vi "P6 main start.vi"() -> ()   [LabVIEW 2016]
doc: "This is the main vi for the C(T) experiment, which measures the capacitance of a ferroelectric capacitor for a defined set of temperatures.\n\nPaul K Dixon\nPhysics 350\nCSUSB Physics"
uses:
  globals/C(T) global variables.vi
  C(T) subvis/temp control/globals/temp control global variables.vi
panel:
  in  "Def Set":dbl=30.0 caption="Default Setpoint (C)" format="%.2f"
  in  "Forced Stop":bool
  # "C(T) Experiment Main"
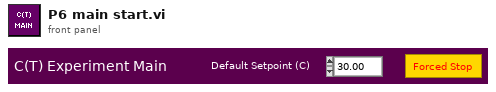
[diagram p1: front panel]
types:
  T1 = typedef "control parameters.ctl" = cluster{"Setpoint":dbl, "Control bandwidth":dbl, "Settle bandwidth":dbl, "Integral time":dbl, "Int\non":bool, "Derivative time":dbl, "Der\non":bool, "Settle time":dbl}
  T2 = cluster{"N cycles for averaging":i32, "N points per measurment":i32, "Measurment time interval":dbl}
  T3 = cluster{"N cycles for averaging":i32, "N points per measurement":i32, "Measurment time interval":dbl}
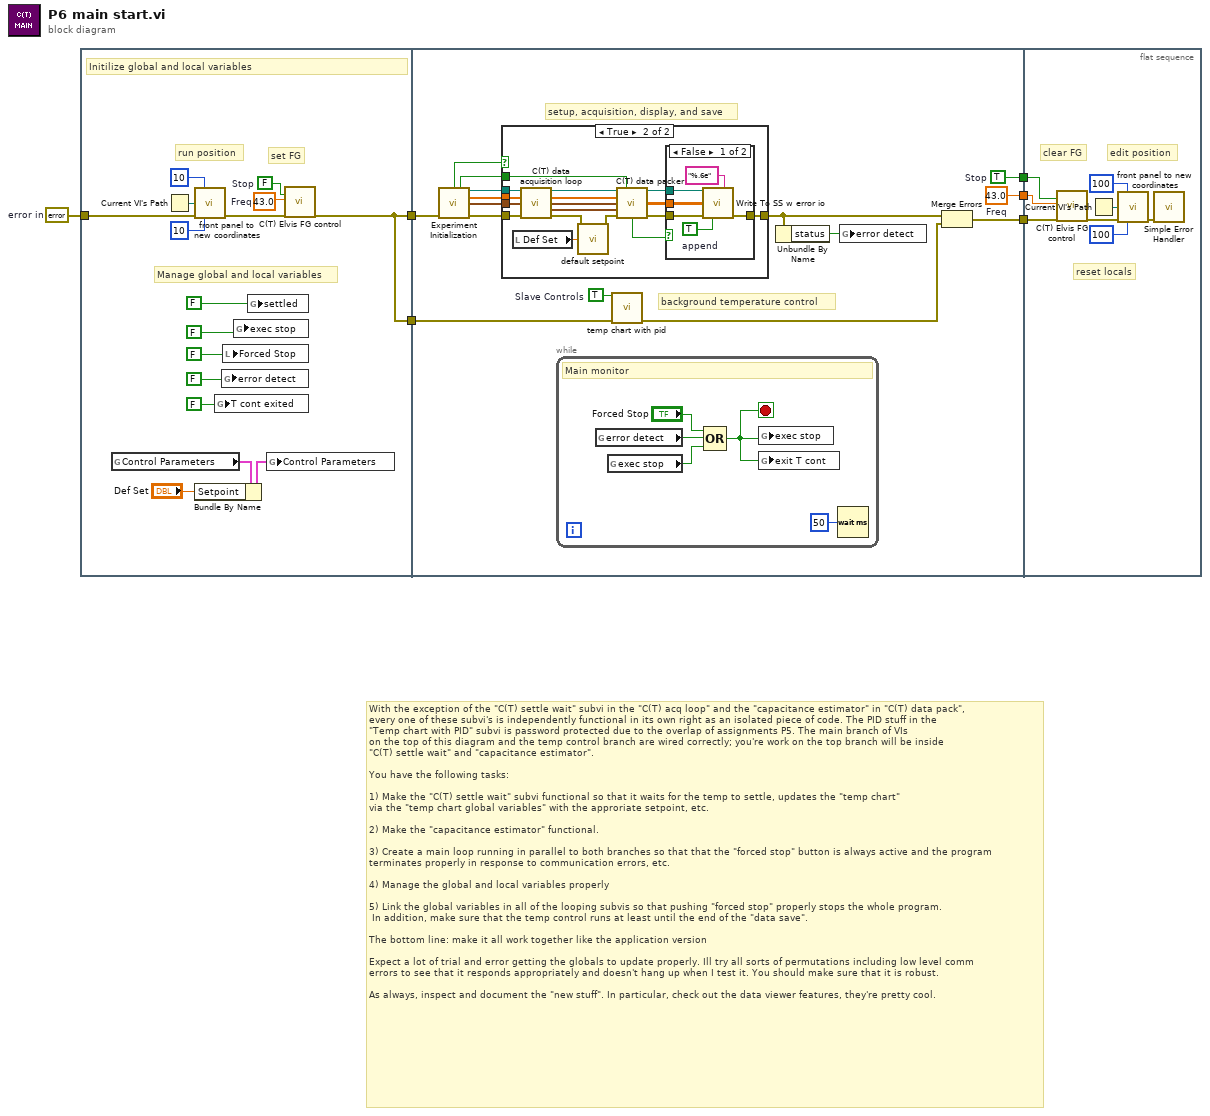
[diagram p0: block diagram]
diagram:
  w4 = errorcluster {"status"=FALSE, "code"=0, "source"=""}  # error in
  # "With the exception of the \"C(T) settle wait\" subvi in the \"C(T) acq loop\" and the \"capacitance estimator\" in \"C(T) data pack\",\nevery one of these subvi's is independently functional in its own right as an isolated piece of code. The PID stuff in the \n\"Temp chart with PID\" subvi is password protected due to the overlap of assignments P5. The main branch of VIs\non the top of this diagram and the temp control branch are wired correctly; you're work on the top branch will be inside \n\"C(T) settle wait\" and \"capacitance estimator\".\n\nYou have the following tasks:\n\n1) Make the \"C(T) settle wait\" subvi functional so that it waits for the temp to settle, updates the \"temp chart\" \nvia the \"temp chart global variables\" with the approriate setpoint, etc.\n\n2) Make the \"capacitance estimator\" functional.\n\n3) Create a main loop running in parallel to both branches so that that the \"forced stop\" button is always active and the program\nterminates properly in response to communication errors, etc.\n\n4) Manage the global and local variables properly \n\n5) Link the global variables in all of the looping subvis so that pushing \"forced stop\" properly stops the whole program.\n In addition, make sure that the temp control runs at least until the end of the \"data save\".\n\nThe bottom line: make it all work together like the application version\n\nExpect a lot of trial and error getting the globals to update properly. Ill try all sorts of permutations including low level comm \nerrors to see that it responds appropriately and doesn't hang up when I test it. You should make sure that it is robust.\n\nAs always, inspect and document the \"new stuff\". In particular, check out the data viewer features, they're pretty cool."
  n1 = flat-sequence {
    tunnel: [w15] -> w6
    tunnel: [w15] -> w5
    tunnel: w4 -> [w19]
    tunnel: w6 -> [w37]
    tunnel: w5 -> [w35]
    tunnel: [w32] -> w3
    tunnel: [w31] -> w2
    tunnel: [w30] -> w1
    tunnel: w3 -> [w70]
    tunnel: w2 -> [w69]
    tunnel: w1 -> [w68]
    frame #0 {
      w17 = 43.0  # Freq
      w18 = FALSE  # Stop
      # "Manage global and local variables"
      # "set FG"
      # "run position"
      # "Initilize global and local variables"
      n2 = global read "temp control global variables.vi" "Control Parameters"() -> (w14:T1)
      n3 = Current VI's Path() -> (path=w20:path)
      n4 = call "front panel to new coordinates.vi"("new top"=i16 10, "path"=w20, "error in (no error)"=w19, "new left"=i16 10) -> ("error out"=w16:errorcluster)  [unwired: 11 out]
      n5 = Bundle By Name(cluster=w14, "Setpoint"="Def Set") -> (w12:T1)
      n6 = global write "temp control global variables.vi" "T cont exited"(FALSE ("T cont exited")) -> ()
      n7 = global write "C(T) global variables.vi" "error detect"(FALSE ("error detect")) -> ()
      n8 = local write "Forced Stop"(FALSE ("Forced Stop")) -> ()
      n9 = global write "C(T) global variables.vi" "exec stop"(FALSE ("exec stop")) -> ()
      n10 = global write "temp control global variables.vi" "settled"(FALSE ("settled")) -> ()
      n11 = global write "temp control global variables.vi" "Control Parameters"(w12) -> ()
      n12 = call "C(T) Elvis FG control.vi"("Stop"=w18, "Frequency (Hz)"=w17, "error in"=w16) -> ("error out"=w15:errorcluster)  [unwired: 15 in, 1 out]
    }
    frame #1 {
      w30 = 43.0  # Freq
      w31 = TRUE  # Stop
      w36 = TRUE  # Slave Controls
      # "setup, acquisition, display, and save"
      # "background temperature control"
      n13 = call "Experiment Initialization.vi"("error in (no error)"=w37) -> ("Go Forward"=w24:bool, "Auto Launch Data Viewer at End"=w25:bool, "data file path out"=w28:path, "Temp Array"=w27:dbl[], "Timing Control Parameters out"=w26:T2, "error out"=w29:errorcluster)  [unwired: 3 in, 6 out]
      n14 = case shown="True" w24 {
        tunnel: w29 -> [w43 w60]
        tunnel: w28 -> [_ w59]
        tunnel: w27 -> [_ w58]
        tunnel: w26 -> [_ w57]
        tunnel: w25 -> [_ w56]
        tunnel: [w43 w48] -> w34
        frame False {
        }
        frame True {
          n15 = local read "Def Set"() -> (w46:dbl)
          n16 = call "C(T) data acquisition loop.vi"("Path in"=w59, "Temp Array In"=w58, "Timing Control Parameters In"=w57, "error in"=w60) -> ("Path out"=w54:path, "Temp Array Out"=w52:dbl[], "Timing Control Parameters Out"=w51:T3, "Normalized Data Out"=w50:waveform(dbl)[], "error out"=w45:errorcluster)  [unwired: 1 in, 6 out]
          n17 = call "default setpoint.vi"("error in (no error)"=w45, "Def Set"=w46) -> ("error out"=w44:errorcluster)  [unwired: 13 in]
          n18 = call "C(T) data packer.vi"("Path in"=w54, "launch viewer"=w56, "Temp Array In"=w52, "Timing Control Parameters In"=w51, "Data In"=w50, "error in"=w44) -> ("Path out"=w53:path, "data spreadsheet"=w49:dbl[][], "no save out"=w47:bool, "error out"=w55:errorcluster)  [unwired: 6 out]
          n19 = case shown="False" w47 {
            tunnel: w55 -> [w66 w67]
            tunnel: w53 -> [w65 _]
            tunnel: w49 -> [w64 _]
            tunnel: [w61 w67] -> w48
            frame False {
              w62 = TRUE  # append
              n20 = call "Write To SS w error io.vi"("file path (dialog if empty)"=w65, "format (%.3f)"="%.6e", "2D data"=w64, "error in"=w66, "append to file? (new file:F)"=w62) -> ("error out"=w61:errorcluster)  [unwired: 4 in, 6 out]
            }
            frame True {
            }
          }
        }
      }
      n21 = while {
        stop <- w38 stop-if-true
        # "Main monitor"
        n22 = global read "C(T) global variables.vi" "error detect"() -> (w40:bool)
        n23 = global read "C(T) global variables.vi" "exec stop"() -> (w39:bool)
        n24 = Compound Arithmetic op=OR("Forced Stop", w40, w39) -> (w38:bool)
        n25 = global write "C(T) global variables.vi" "exec stop"(w38) -> ()
        n26 = global write "temp control global variables.vi" "exit T cont"(w38) -> ()
        n27 = Wait (ms)(milliseconds to wait=u32 50) -> ()  [unwired: 1 out]
      }
      n28 = call "temp chart with pid.vi"("Slave Controls"=w36, "error in"=w35) -> ("error out"=w33:errorcluster)  [unwired: 3 in, 10 out]
      n29 = Unbundle By Name(w34) -> ("status"=w23:bool)
      n30 = global write "C(T) global variables.vi" "error detect"(w23) -> ()
      n31 = Merge Errors(w34, w33) -> (w32:errorcluster)
    }
    frame #2 {
      # "clear FG"
      # "reset locals"
      # "edit position"
      n32 = call "C(T) Elvis FG control.vi"("Stop"=w69, "Frequency (Hz)"=w68, "error in"=w70) -> ("error out"=w71:errorcluster)  [unwired: 15 in, 1 out]
      n33 = Current VI's Path() -> (path=w75:path)
      n34 = call "front panel to new coordinates.vi"("new top"=i16 100, "path"=w75, "error in (no error)"=w71, "new left"=i16 100) -> ("error out"=w72:errorcluster)  [unwired: 11 out]
      n35 = call <vilib>:"Simple Error Handler.vi"("error in (no error)"=w72) -> ()  [unwired: 1 in, 8 out]
    }
  }
